vi "Update Map History.vi"(8 "error in (no error)":errorcluster, 9 "Y":dbl, 10 "X":dbl, 11 "FormulaG App in":refnum<class "FormulaG App.lvclass">) -> (0 "error out":errorcluster, 2 "XY Graph":cluster{dbl[], dbl[]}[](array[cluster]), 3 "FormulaG App out":refnum<class "FormulaG App.lvclass">)   [LabVIEW 2020, in "FormulaG.lvlib" / "FormulaG App.lvclass"]
uses:
  FormulaG App.lvclass
  FormulaG App.lvclass/FormulaG App.ctl
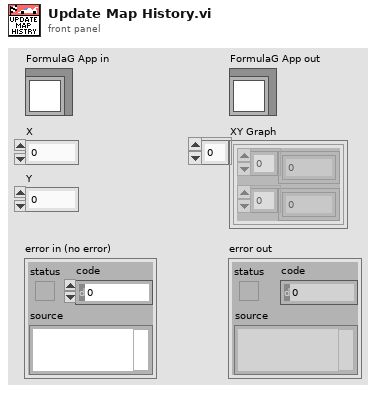
[diagram p1: front panel]
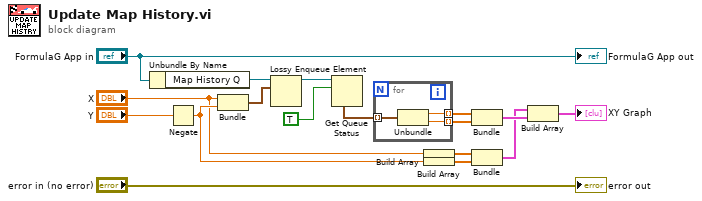
[diagram p0: block diagram]
diagram:
  n1 = Unbundle By Name("FormulaG App in") -> ("Map History Q"=w4:refnum<queue>)
  n2 = Negate(x="Y") -> (-x=w13:dbl)
  n3 = Bundle("X"="X", w13) -> (w16:cluster{"X":dbl, dbl})  [unwired: 1 in]
  n4 = Lossy Enqueue Element(queue=w4, element=w16) -> (queue out=w15:refnum<queue>)  [unwired: 1 in, 3 out]
  n5 = Get Queue Status(queue=w15, return elements? (F)=TRUE) -> (elements=w12:cluster{dbl, dbl}[])  [unwired: 1 in, 7 out]
  n6 = for {
    tunnel: w12 -> [w20] mode=indexing
    tunnel: [w19] -> w9 mode=indexing
    tunnel: [w18] -> w8 mode=indexing
    n7 = Unbundle(w20) -> (w19:dbl, w18:dbl)
  }
  n8 = Build Array("X") -> (w11:dbl[])
  n9 = Build Array(w13) -> (w10:dbl[])
  n10 = Bundle(w9, w8) -> (w7:cluster{dbl[], dbl[]})  [unwired: 1 in]
  n11 = Bundle(w11, w10) -> (w6:cluster{dbl[], dbl[]})  [unwired: 1 in]
  n12 = Build Array(w6, w7) -> (→"XY Graph":cluster{dbl[], dbl[]}[])
  "error out" <- "error in (no error)"
  "FormulaG App out" <- "FormulaG App in"
